vi "test-AttrMap-SetValue.vi"(8 "error in (no error)":errorcluster, 11 "TestCase in":refnum<class "MyTestCase.lvclass">) -> (0 "error out":errorcluster, 3 "TestCase out":refnum<class "MyTestCase.lvclass">)   [LabVIEW 2019, in "MyTestCase.lvclass"]
uses:
  MyTestCase.lvclass
  <vilib>/addons/_JKI Toolkits/VI Tester/TestCase.llb/TestCase.lvclass
  src/lv-apt-json-file.lvlib
  C:/Program Files (x86)/National Instruments/LabVIEW 2019/vi.lib/addons/_JKI Toolkits/VI Tester/TestCase.llb/TestCase.lvclass
panel:
  in  "Tree":string(tree)
  out "OrignKey":string
  out "Variant":variant
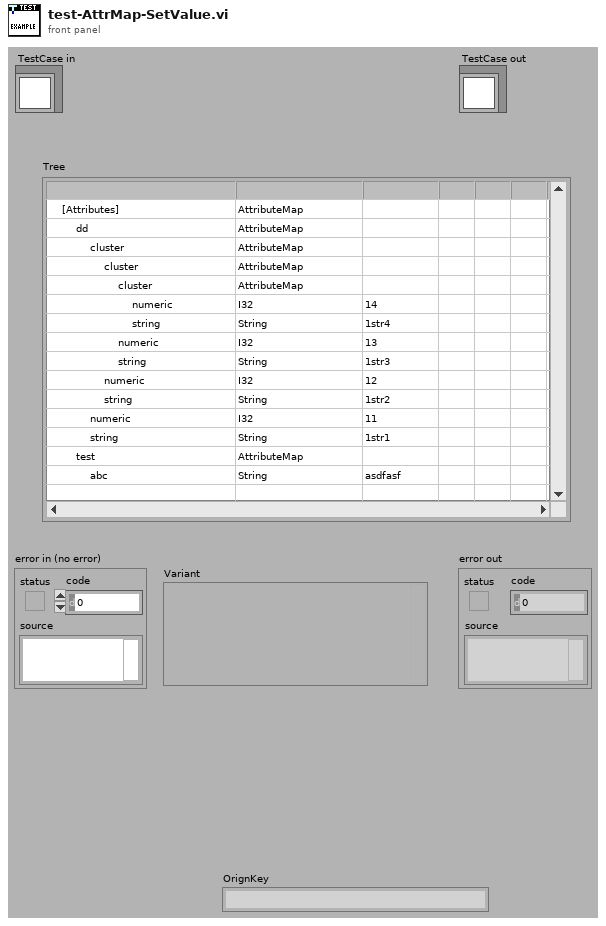
[diagram p1: front panel]
types:
  T1 = cluster{"nUmeric":i32, "string":string, "Cluster":cluster{"numeric":i32, "string":string, "cluster":cluster{"numeric":i32, "string":string, "cluster":cluster{"numeric":i32, "string":string}}}}
  T2 = typedef "lv-apt-json-file.lvlib/Def-AttrMap.ctl" = cluster{"Map":variant}
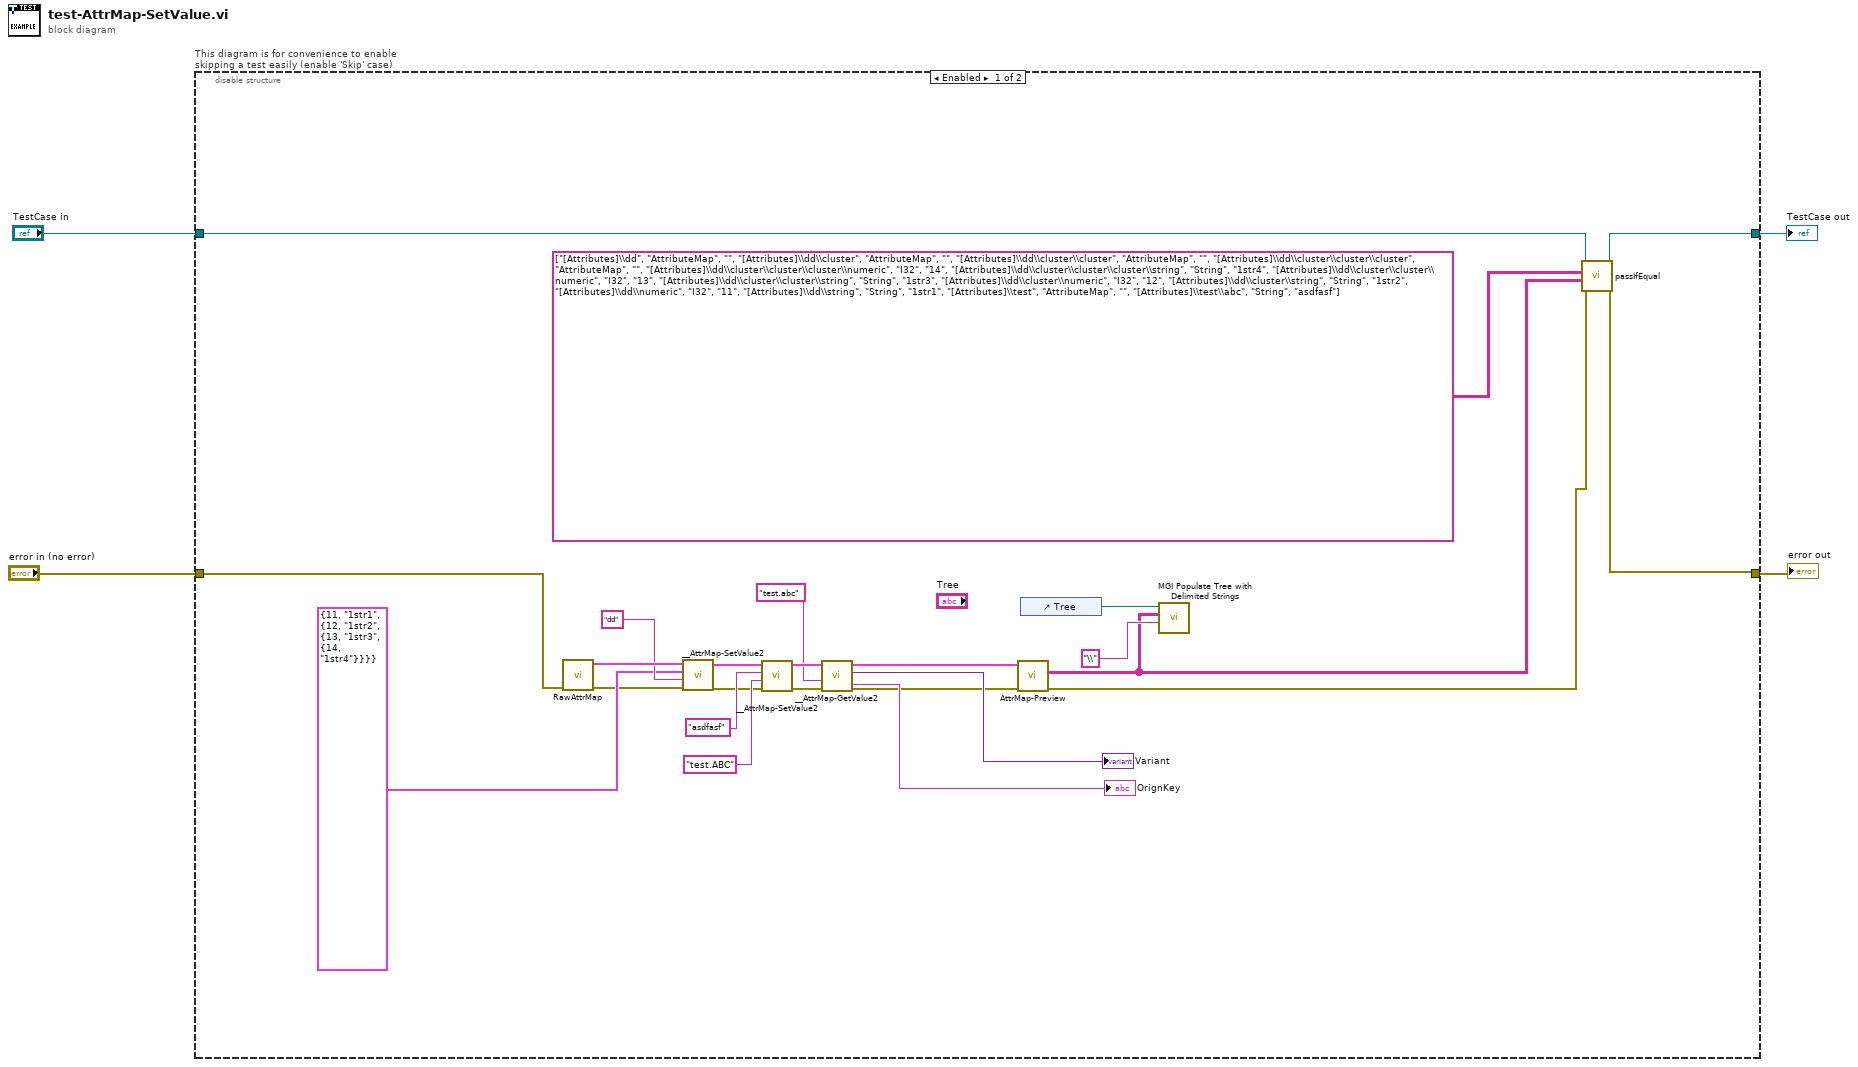
[diagram p0: block diagram]
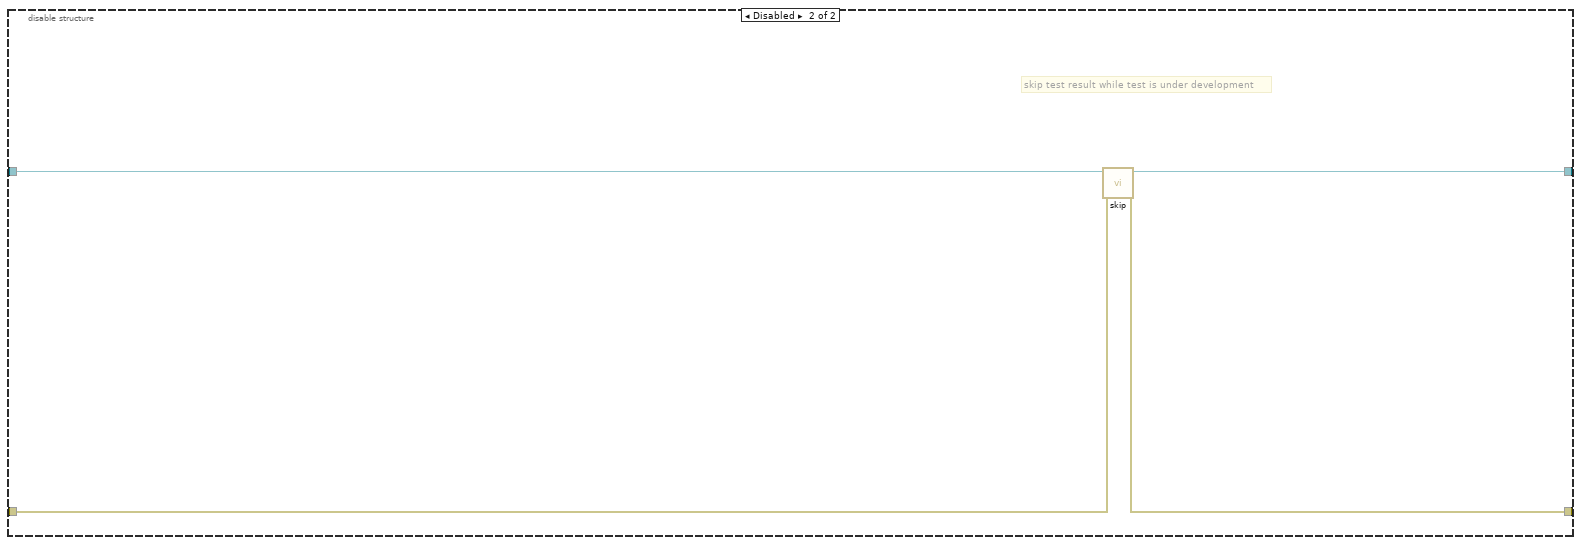
[diagram p2: hidden frame]
diagram:
  n1 = disable-structure "This diagram is for convenience to enable skipping a test easily (enable 'Skip' case)" shown="Enabled" {
    disable-tunnel: "TestCase in" -> [w27 w31]
    disable-tunnel: [w26 w29] -> w1
    disable-tunnel: [w25 w30] -> w3
    disable-tunnel: "error in (no error)" -> [w10 w28]
    frame Enabled {
      n2 = call "RawAttrMap.vi"() -> ("AttrMap"=w17:T2)  [unwired: 11 in]
      n3 = call "__AttrMap-SetValue2.vi"("error in (no error)"=w10, "Key"="dd", "Value"=T1 {"nUmeric"=11, "string"="1str1", "Cluster"={"numeric"=12, "string"="1str2", "cluster"={"numeric"=13, "string"="1str3", "cluster"={"numeric"=14, "string"="1str4"}}}} ("Cluster"), "AttrMap in"=w17) -> ("error out"=w15:errorcluster, "AttrMap out"=w16:T2)  [unwired: 6 in]
      n4 = call "__AttrMap-SetValue2.vi"("error in (no error)"=w15, "Key"="test.ABC", "Value"="asdfasf", "AttrMap in"=w16) -> ("error out"=w18:errorcluster, "AttrMap out"=w24:T2)  [unwired: 6 in]
      n5 = call "__AttrMap-GetValue2.vi"("error in (no error)"=w18, "Key"="test.abc", "AttrMap in"=w24) -> ("error out"=w11:errorcluster, "VAttributes"=→"Variant":variant, "AttrMap out"=w12:T2, "OrignKey"=→"OrignKey":string)  [unwired: 4 in, 1 out]
      n6 = call "AttrMap-Preview.vi"("error in (no error)"=w11, "AttrMap in"=w12) -> ("error out"=w9:errorcluster, "table"=w5:string[][])  [unwired: 7 in, 1 out]
      n7 = control-ref of="Tree"() -> (w8:refnum<vi>)
      n8 = call <userlib>:"MGI Populate Tree with Delimited Strings.vi"("Delimiter"="\\", "Items (Delimited)"=w5, "Tree Control"=w8) -> ()  [unwired: 6 in, 3 out]
      n9 = call-dynamic "passIfEqual.vi"("error in (no error)"=w9, "y"=w5, "x"=string[][] [["[Attributes]\\dd", "AttributeMap", ""], ["[Attributes]\\dd\\cluster", "AttributeMap", ""], ["[Attributes]\\dd\\cluster\\cluster", "AttributeMap", ""], ["[Attributes]\\dd\\cluster\\cluster\\cluster", "AttributeMap", ""], ["[Attributes]\\dd\\cluster\\cluster\\cluster\\numeric", "I32", "14"], ["[Attributes]\\dd\\cluster\\cluster\\cluster\\string", "String", "1str4"], ["[Attributes]\\dd\\cluster\\cluster\\numeric", "I32", "13"], ["[Attributes]\\dd\\cluster\\cluster\\string", "String", "1str3"], ["[Attributes]\\dd\\cluster\\numeric", "I32", "12"], ["[Attributes]\\dd\\cluster\\string", "String", "1str2"], ["[Attributes]\\dd\\numeric", "I32", "11"], ["[Attributes]\\dd\\string", "String", "1str1"], ["[Attributes]\\test", "AttributeMap", ""], ["[Attributes]\\test\\abc", "String", "asdfasf"]] ("table"), "TestCase in"=w27) -> ("error out"=w25:errorcluster, "TestCase out"=w26:refnum<class "MyTestCase.lvclass">)  [unwired: 6 in]
    }
    frame Disabled {
      # "skip test result while test is under development"
      n10 = call <vilib>:"skip.vi"("error in (no error)"=w28, "TestCase in"=w31) -> ("error out"=w30:errorcluster, "TestCase out"=w29:refnum<class "MyTestCase.lvclass">)  [unwired: 8 in]
    }
  }
  "error out" <- w3
  "TestCase out" <- w1
